vi "OpenConnection.vi"(8 "error in (no error)":errorcluster, 10 "MongoDB Connection String":string) -> (0 "error out":errorcluster, 3 "MongoDB-Client out":refnum<class "MongoDB-Client.lvclass">)   [LabVIEW 2016, in "MongoDB-Client.lvlib" / "MongoDB-Client.lvclass"]
uses:
  MongoDB-Client.lvclass
  D:/Users/blume/Desktop/LV/MongoDB-Driver/MLV DLLs/MongoLabVIEW.dll
  LV/MongoDB-Driver/MLV DLLs/MongoLabVIEW.dll
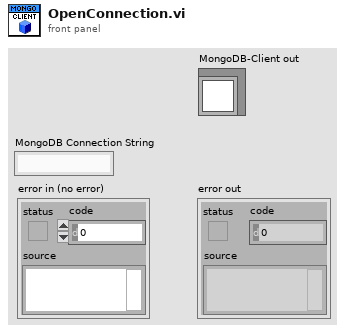
[diagram p1: front panel]
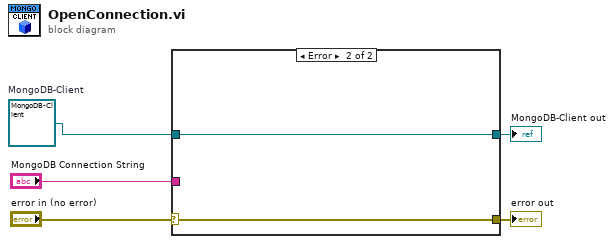
[diagram p0: block diagram]
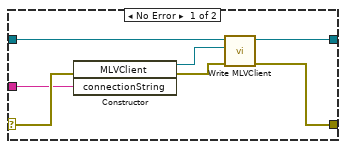
[diagram p2: hidden frame]
diagram:
  w1 = refnum<class "MongoDB-Client.lvclass"> refnum  # MongoDB-Client
  n1 = case shown="Error" "error in (no error)" {
    selector: "error in (no error)" -> [w12 w14]
    tunnel: [w8 w14] -> w4
    tunnel: [w10 w13] -> w3
    tunnel: "MongoDB Connection String" -> [w11 _]
    tunnel: w1 -> [w6 w13]
    frame No Error {
      n2 = constructor class="MLVClient"(error in=w12, "connectionString"=w11) -> (reference out=w7:refnum<k24>, error out=w9:errorcluster)  [unwired: 2 in, 2 out]
      n3 = call "Write MLVClient.vi"("error in (no error)"=w9, "MLVClient"=w7, "MongoDB-Client in"=w6) -> ("error out"=w8:errorcluster, "MongoDB-Client out"=w10:refnum<class "MongoDB-Client.lvclass">)  [unwired: 7 in]
    }
    frame Error {
    }
  }
  "error out" <- w4
  "MongoDB-Client out" <- w3
